vi "Read Value.vi"(8 "error in (no error)":errorcluster, 11 "DBL Result in":refnum<class "DBL Payload.lvclass">) -> (0 "error out":errorcluster, 2 "Value":dbl, 3 "DBL Result out":refnum<class "DBL Payload.lvclass">)   [LabVIEW 2015, in "DBL Payload.lvclass"]
uses:
  DBL Payload.lvclass
  DBL Payload.lvclass/DBL Payload.ctl
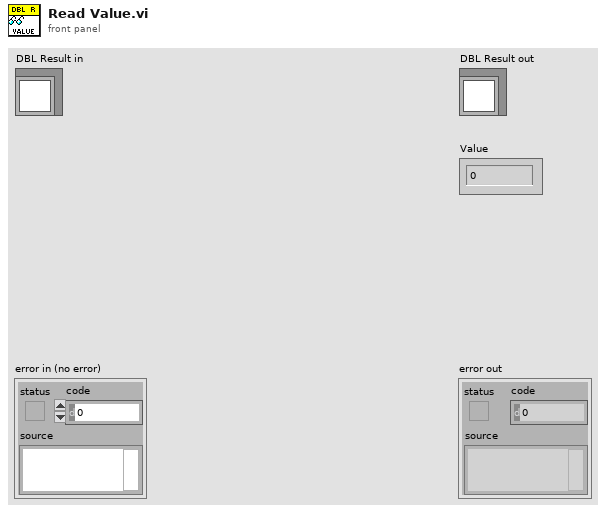
[diagram p1: front panel]
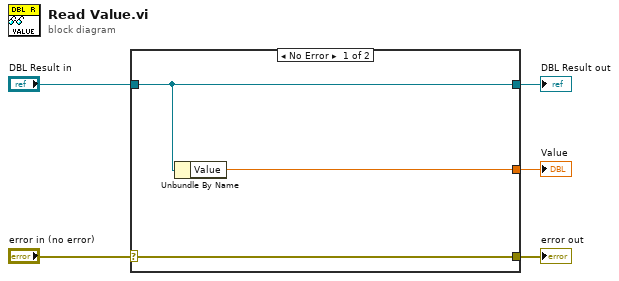
[diagram p0: block diagram]
diagram:
  n1 = case shown="No Error" "error in (no error)" {
    selector: "error in (no error)" -> [w8 w9]
    tunnel: [w8 w9] -> w4
    tunnel: [w7 w10] -> w2
    tunnel: "DBL Result in" -> [w7 w10]
    tunnel: [w6 _] -> w1
    frame No Error {
      n2 = Unbundle By Name(w7) -> ("Value"=w6:dbl)
    }
    frame Error {
    }
  }
  "error out" <- w4
  "DBL Result out" <- w2
  "Value" <- w1
